vi "Drive Controller Interactive Check.vi"(8 "Interactive Command In":T1 {"Auto Path Data"."Commands"."System" items=["FLoating Intake"=2, "Carriage Intake"=1, "Elevator"=0]; "Auto Path Data"."Commands"."System Selection" items=["FLoating Intake"=2, "Carriage Intake"=1, "Elevator"=0]}, 9 "Default Command":T1 {"Auto Path Data"."Commands"."System" items=["FLoating Intake"=2, "Carriage Intake"=1, "Elevator"=0]; "Auto Path Data"."Commands"."System Selection" items=["FLoating Intake"=2, "Carriage Intake"=1, "Elevator"=0]}, 11 "Buttons":cluster{"Execute Cmd":bool, "Abort Cmd":bool}) -> (1 "Interactive Command Out":T1 {"Auto Path Data"."Commands"."System" items=["FLoating Intake"=2, "Carriage Intake"=1, "Elevator"=0]; "Auto Path Data"."Commands"."System Selection" items=["FLoating Intake"=2, "Carriage Intake"=1, "Elevator"=0]}, 2 "Trace String":string, 3 "Schedule":bool)   [LabVIEW 2018]
doc: "Check the Execute and Abort buttons and choose the data and trace string."
uses:
  Drive Setpoints.ctl
  Drive Operations.ctl
  Support Code/Path Data.ctl
  Support Code/Availible Command systems for auto.ctl
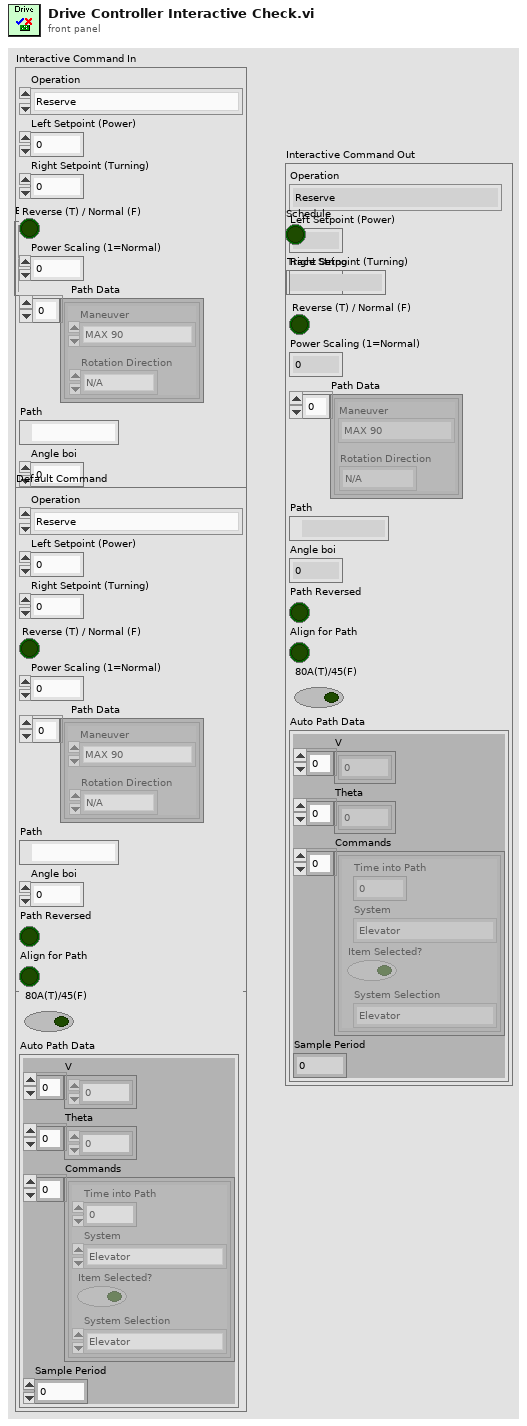
[diagram p1: front panel]
types:
  T1 = typedef "Drive Setpoints.ctl" = cluster{"Operation":T2, "Left Setpoint (Power)":dbl, "Right Setpoint (Turning)":dbl, "Reverse (T) / Normal (F)":bool, "Power Scaling (1=Normal) ":dbl, "Path Data":T3, "Path":path, "Angle boi":dbl, "Path Reversed":bool, "Align for Path":bool, "80A(T)/45(F)":bool, "Auto Path Data":cluster{"V":dbl[], "Theta":dbl[], "Commands":cluster{"Time into Path":dbl, "System":T4, "Item Selected?":bool, "System Selection":T4}[], "Sample Period":dbl}}
  T2 = typedef "Drive Operations.ctl" = enum16{"Reserve", "Read Current", "Immediate", "J-Turn", "Play Back From Log", "Auto-Align"}
  T3 = typedef "Path Data.ctl" = cluster{"Maneuver":enum16{"MAX 90", "MAX 180", "Turn to Home", "Turn to Rocket", "Auto-Align", "Turn to ..."}, "Rotation Direction":enum16{"N/A", "Right", "Left"}}[]
  T4 = typedef "Availible Command systems for auto.ctl" = u16
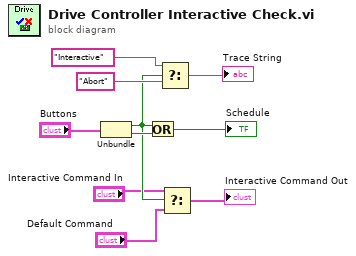
[diagram p0: block diagram]
diagram:
  n1 = Unbundle("Buttons") -> ("Execute Cmd"=w6:bool, "Abort Cmd"=w7:bool)
  n2 = Or(x=w6, y=w7) -> (x .or. y?=→"Schedule":bool)
  n3 = Select(t="Interactive", s=w6, f="Abort") -> (s? t:f=→"Trace String":string)
  n4 = Select(t="Interactive Command In", s=w6, f="Default Command") -> (s? t:f=→"Interactive Command Out":T1)
